vi "oa_Get Resampled Signal Cycle by Cycle (N Channels).vi"(0 "resampled signal":cluster{"r0":dbl, "dr":dbl, "Y":dbl[]}[](array[cluster]) {"r0" format="%.2p"; "dr" format="%.2p"; "Y" format="%.2f"}, 1 "reset?":bool=TRUE, 11 "error in":errorcluster) -> (4 "resampled signal out":cluster{"r0":dbl, "dr":dbl, "Y":dbl[]}[][](array[cluster]) {"r0" format="%.2p"; "dr" format="%.2p"; "Y" format="%.2f"}, 15 "error out":errorcluster)   [LabVIEW 2017, in "SoundVib_RefDataProcess.lvlib"]
uses:
  <vilib>/addons/Sound and Vibration/Order Analysis/Referece Data Processing/SoundVib_RefDataProcess.lvlib
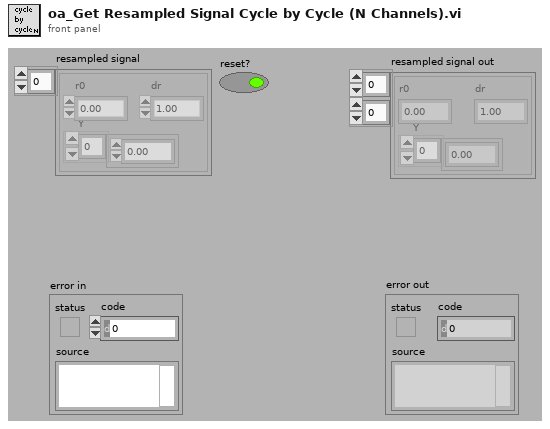
[diagram p1: front panel]
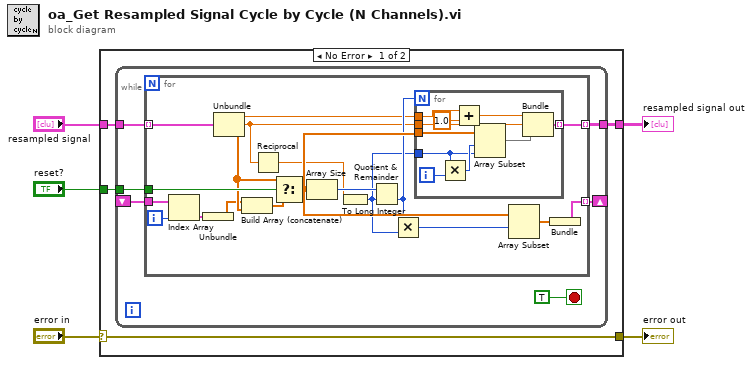
[diagram p0: block diagram]
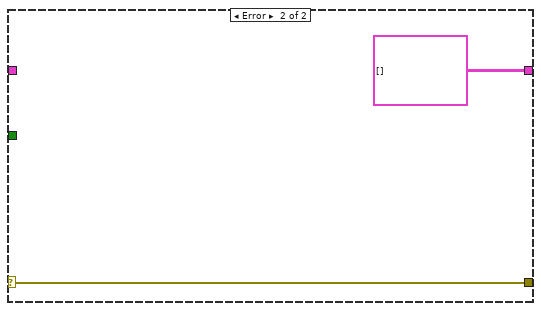
[diagram p2: hidden frame]
diagram:
  n1 = case shown="No Error" "error in" {
    selector: "error in" -> [w8 w46]
    tunnel: [w8 w46] -> w3
    tunnel: "resampled signal" -> [w9 _]
    tunnel: "reset?" -> [w7 _]
    tunnel: [w6 cluster{dbl, "dr":dbl, dbl[]}[][] []] -> w1
    frame No Error {
      n2 = while {
        tunnel: w9 -> [w15]
        shift-right: [w11] -> _
        shift-left: _ -> [w12]
        tunnel: w7 -> [w13]
        tunnel: [w10] -> w6
        stop <- TRUE stop-if-true
        n3 = for {
          tunnel: w15 -> [w34] mode=indexing
          tunnel: w13 -> [w32]
          tunnel: w12 -> [w19]
          tunnel: [w20] -> w11 mode=indexing
          tunnel: [w22] -> w10 mode=indexing
          i -> [w18]
          n4 = Index Array(array=w19, index=w18) -> (element=w17:cluster{dbl[]})
          n5 = Unbundle(w17) -> (w16:dbl[])
          n6 = Unbundle(w34) -> ("r0"=w25:dbl, "dr"=w24:dbl, "Y"=w31:dbl[])
          n7 = Build Array (concatenate)(w16, w31) -> (w30:dbl[])
          n8 = Reciprocal(x=w24) -> (1/x=w23:dbl)
          n9 = Select(t=w31, s=w32, f=w30) -> (s? t:f=w27:dbl[])
          n10 = Array Size(array=w27) -> (size(s)=w33:i32)
          n11 = To Long Integer(number=w23) -> (32bit integer=w21:i32)
          n12 = Quotient & Remainder(x=w33, y=w21) -> (floor(x/y)=w26:i32)  [unwired: 1 out]
          n13 = Multiply(x=w26, y=w21) -> (x*y=w29:i32)
          n14 = for {
            N: w26 -> [_]
            tunnel: w27 -> [w44]
            tunnel: w21 -> [w37]
            tunnel: w24 -> [w40]
            tunnel: w25 -> [w38]
            tunnel: [w35] -> w22 mode=indexing
            i -> [w43]
            n15 = Multiply(x=w37, y=w43) -> (x*y=w42:i32)
            n16 = Add(x=w38, y=1.0) -> (x+y=w39:dbl)
            n17 = Array Subset(array=w44, index=w42, length=w37) -> (w41:dbl[])
            n18 = Bundle(w39, "dr"=w40, w41) -> (w35:cluster{dbl, "dr":dbl, dbl[]})  [unwired: 1 in]
          }
          n19 = Array Subset(array=w27, index=w29) -> (w28:dbl[])  [unwired: 1 in]
          n20 = Bundle(w28) -> (w20:cluster{dbl[]})  [unwired: 1 in]
        }
      }
    }
    frame Error {
    }
  }
  "error out" <- w3
  "resampled signal out" <- w1
